vi "CreateHardwareActionQueues.vi"(8 "Error In":errorcluster) -> (0 "Error Out":errorcluster, 3 "Hardware Action Queues":T1)   [LabVIEW 2012]
uses:
  HardwareActionQueues.ctl
  PXI6229ActionQueueElement.ctl
  PXI6229Action.ctl
  CurrentMeterQueueElement.ctl
  CurrentMeterAction.ctl
  HardwareLogActionQueueElement.ctl
  HardwareLogAction.ctl
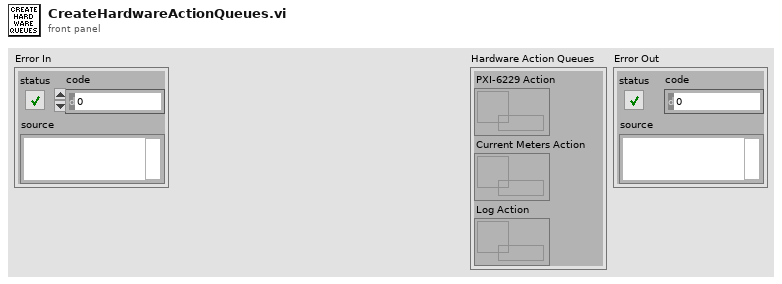
[diagram p1: front panel]
types:
  T1 = typedef "HardwareActionQueues.ctl" = cluster{"PXI-6229 Action":refnum<queue>, "Current Meters Action":refnum<queue>, "Log Action":refnum<queue>}
  T2 = typedef "HardwareLogActionQueueElement.ctl" = cluster{"Action":T3, "Data":variant}
  T3 = typedef "HardwareLogAction.ctl" = enum16{"Initialize", "Clear", "Create", "Log", "Stop", "Shutdown"}
  T4 = typedef "CurrentMeterQueueElement.ctl" = cluster{"Action":T5, "Data":variant}
  T5 = typedef "CurrentMeterAction.ctl" = enum16{"Initialize", "Read", "Simulate", "Error", "Shutdown"}
  T6 = typedef "PXI6229ActionQueueElement.ctl" = cluster{"Action":T7, "Data":variant}
  T7 = typedef "PXI6229Action.ctl" = enum16{"Initialize", "Read", "Simulate", "Error", "Shutdown"}
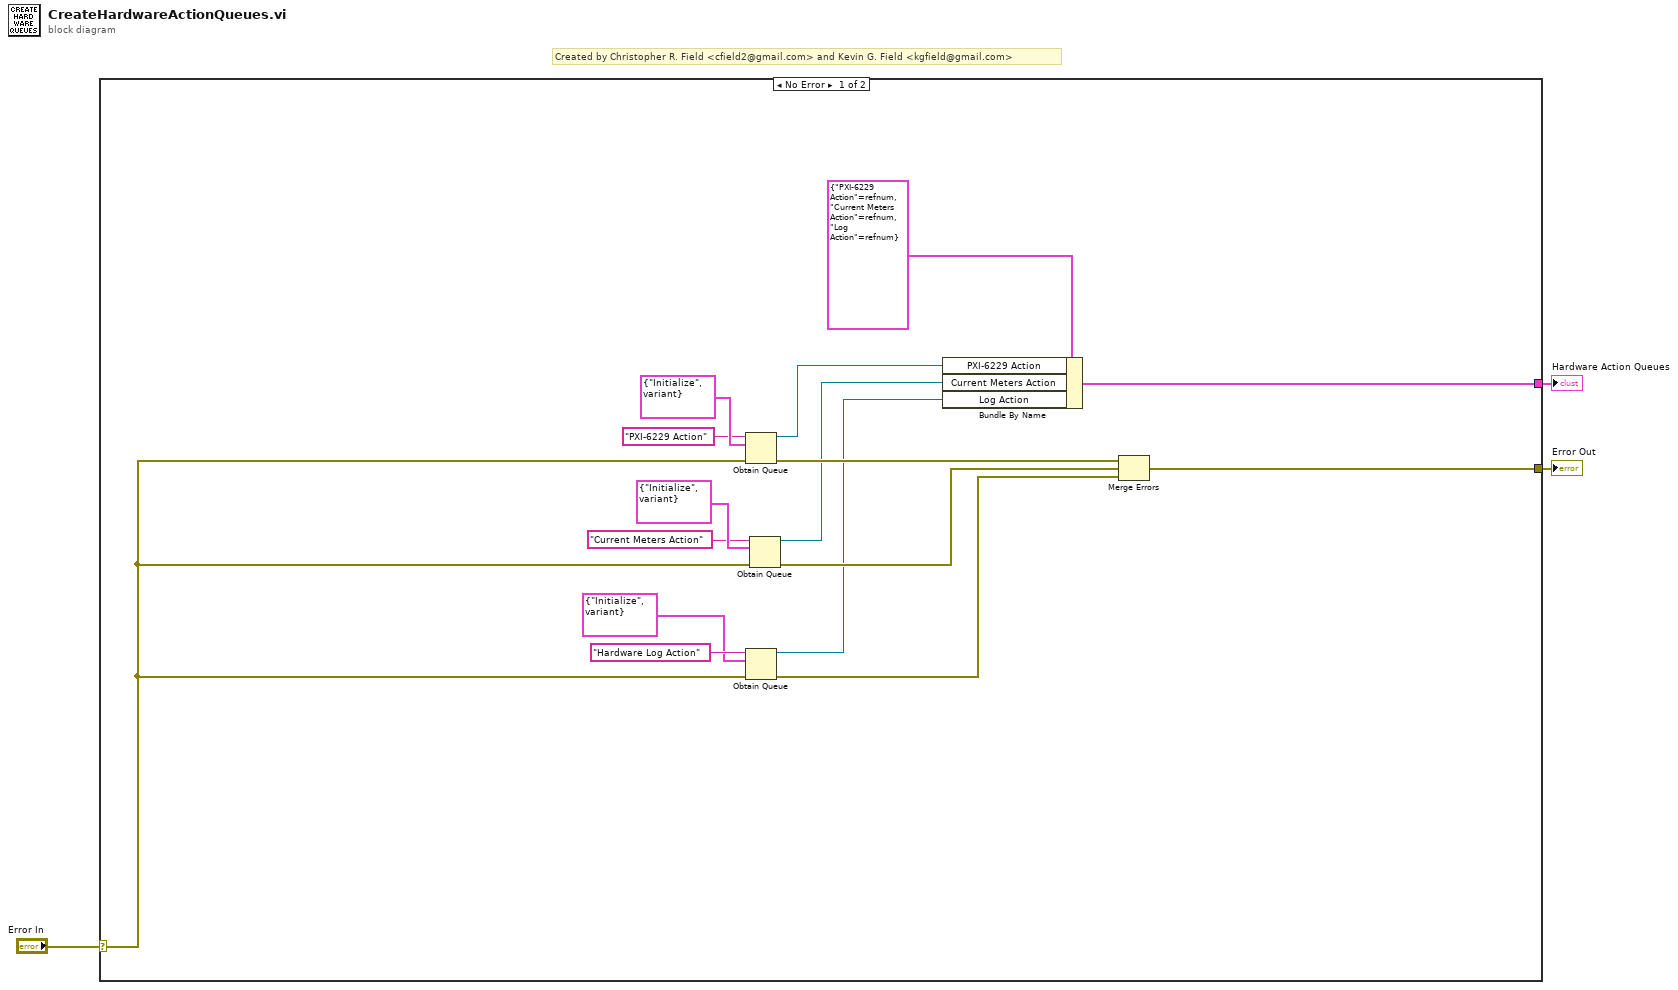
[diagram p0: block diagram]
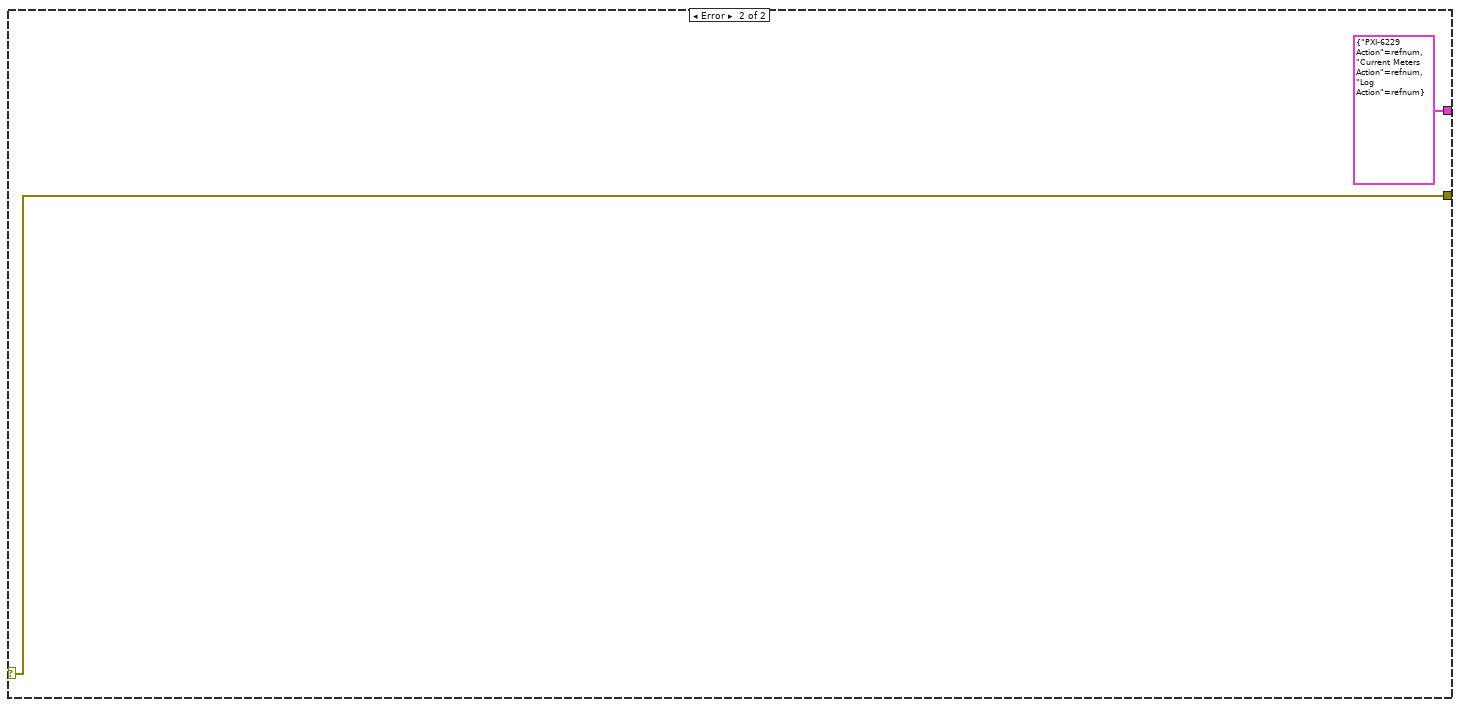
[diagram p2: hidden frame]
diagram:
  # "Created by Christopher R. Field <cfield2@gmail.com> and Kevin G. Field <kgfield@gmail.com>"
  n1 = case shown="No Error" "Error In" {
    selector: "Error In" -> [w14 w21]
    tunnel: [w6 T1 {"PXI-6229 Action"=refnum, "Current Meters Action"=refnum, "Log Action"=refnum} ("Hardware Action Queues")] -> w2
    tunnel: [w5 w21] -> w1
    frame No Error {
      n2 = Obtain Queue(name (unnamed)="PXI-6229 Action", element data type=T6 {"Action"=enum."Initialize", "Data"=variant} ("DAQ Queue Element"), error in (no error)=w14) -> (queue out=w9:refnum<queue>, error out=w13:errorcluster)  [unwired: 2 in, 1 out]
      n3 = Obtain Queue(name (unnamed)="Hardware Log Action", element data type=T2 {"Action"=enum."Initialize", "Data"=variant} ("Hardware Log Queue Element"), error in (no error)=w14) -> (queue out=w7:refnum<queue>, error out=w11:errorcluster)  [unwired: 2 in, 1 out]
      n4 = Obtain Queue(name (unnamed)="Current Meters Action", element data type=T4 {"Action"=enum."Initialize", "Data"=variant} ("Picoamp Meter Queue Element"), error in (no error)=w14) -> (queue out=w8:refnum<queue>, error out=w12:errorcluster)  [unwired: 2 in, 1 out]
      n5 = Bundle By Name(cluster=T1 {"PXI-6229 Action"=refnum, "Current Meters Action"=refnum, "Log Action"=refnum} ("Hardware Action Queues"), "PXI-6229 Action"=w9, "Current Meters Action"=w8, "Log Action"=w7) -> (w6:T1)
      n6 = Merge Errors(w13, w12, w11) -> (w5:errorcluster)
    }
    frame Error {
    }
  }
  "Hardware Action Queues" <- w2
  "Error Out" <- w1
